vi "Read_Battery_System_State_VI.vi"() -> ()   [LabVIEW 2017]
uses:
  <vilib>/Plasmionique/MB Master/MB_Master_TCP/MB_Master_TCP.lvclass
  C:/Program Files (x86)/National Instruments/LabVIEW 2017/vi.lib/Plasmionique/MB Master/MB_Master/MB_Master.lvclass
  <vilib>/Plasmionique/MB Master/MB Master.lvlib
panel:
  out "Status":string
  out "BMS IP Address":string
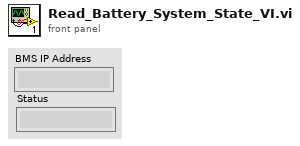
[diagram p1: front panel]
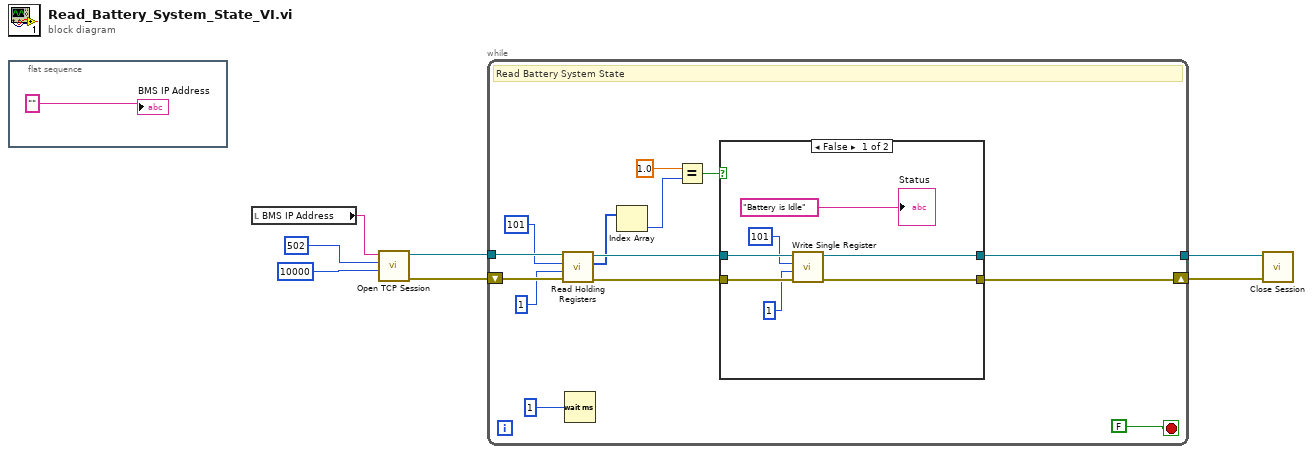
[diagram p0: block diagram]
diagram:
  n1 = flat-sequence {
    frame #0 {
      "BMS IP Address" <- ""
    }
  }
  n2 = local read "BMS IP Address"() -> (w5:string)
  n3 = call <vilib>:"Open TCP Session.vi"("Timeout (10000)"=10000, "Port (502)"=u16 502, "IP Address"=w5) -> ("error out"=w7:errorcluster, "MB_TCP session"=w6:refnum<class "MB_Master_TCP.lvclass">)  [unwired: 7 in]
  n4 = while {
    tunnel: w6 -> [w22]
    shift-right: [w10] -> w1
    shift-left: w7 -> [w21]
    tunnel: [w11] -> w2
    stop <- FALSE stop-if-true
    # "Read Battery System State"
    n5 = call <vilib>:"Read Holding Registers.vi"("error in (no error)"=w21, "quantity"=u16 1, "starting address"=u16 101, "MB session in"=w22) -> ("error out"=w17:errorcluster, "Registers"=w13:u16[], "MB session out"=w18:refnum<class "MB_Master_TCP.lvclass">)  [unwired: 5 in]
    n6 = Wait (ms)(milliseconds to wait=u32 1) -> ()  [unwired: 1 out]
    n7 = Index Array(array=w13) -> (element=w12:u16)  [unwired: 1 in]
    n8 = Equal?(x=1.0, y=w12) -> (x = y?=w15:bool)
    n9 = case shown="False" w15 {
      tunnel: w18 -> [w28 w31]
      tunnel: w17 -> [w27 w30]
      tunnel: [w24 w31] -> w11
      tunnel: [w23 w30] -> w10
      frame False {
        n10 = call <vilib>:"Write Single Register.vi"("error in (no error)"=w27, "value"=u16 1, "address"=u16 101, "MB session in"=w28) -> ("error out"=w23:errorcluster, "MB session out"=w24:refnum<class "MB_Master_TCP.lvclass">)  [unwired: 6 in]
        "Status" <- "Battery is Idle" ("String")
      }
      frame True {
      }
    }
  }
  n11 = call-dynamic "Close Session.vi"("error in (no error)"=w1, "MB TCP session"=w2) -> ()  [unwired: 9 in, 1 out]
